vi "Show Animated Busy Icon with Message.vi"(4 "Animated Busy Icon Control Name (Animated Busy Icon)":string="Animated Busy Icon", 5 "Already active? (F)":bool, 6 "Message Control Name (Message)":string="Message", 7 "Message":string, 9 "Error In":errorcluster, 11 "Target VI reference":refnum<vi>) -> (1 "Error Out":errorcluster)   [LabVIEW 2019]
doc: "This VI passes error in through and ignores it"
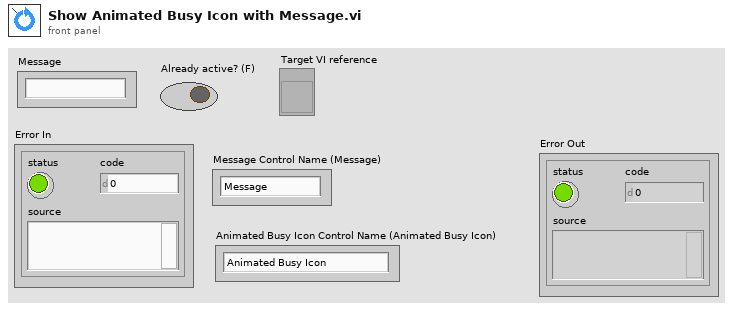
[diagram p1: front panel]
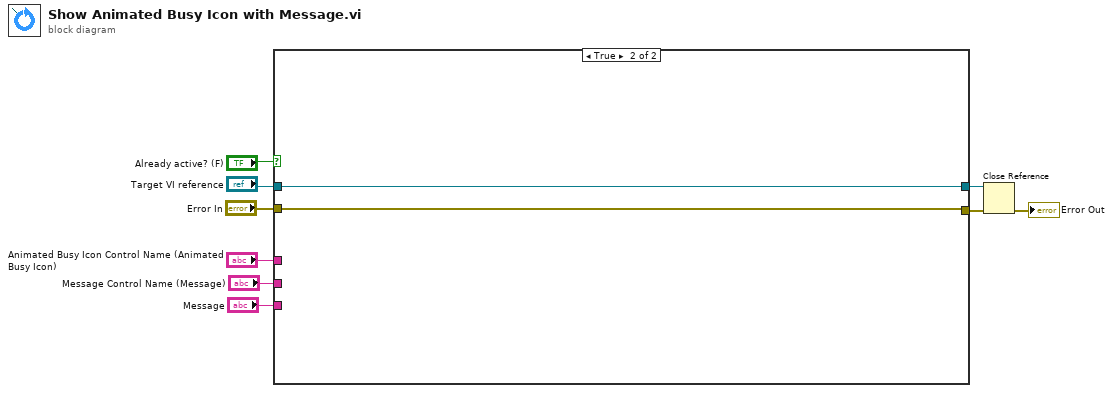
[diagram p0: block diagram]
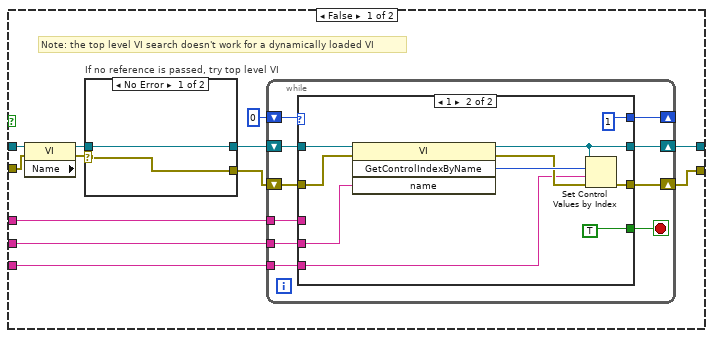
[diagram p2: hidden frame]
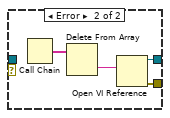
[diagram p3: hidden frame]
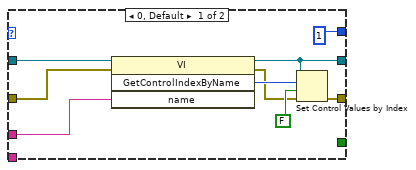
[diagram p4: hidden frame]
diagram:
  n1 = case shown="True" "Already active? (F)" {
    tunnel: [w19 w58] -> w9
    tunnel: [w18 w57] -> w8
    tunnel: "Message Control Name (Message)" -> [w16 _]
    tunnel: "Animated Busy Icon Control Name (Animated Busy Icon)" -> [w15 _]
    tunnel: "Message" -> [w14 _]
    tunnel: "Target VI reference" -> [w13 w58]
    tunnel: "Error In" -> [w10 w57]
    frame False {
      # "Note: the top level VI search doesn't work for a dynamically loaded VI"
      n2 = property class="VI" props=["Name"](reference=w13, error in=w10) -> (reference out=w11:refnum<vi>, error out=w12:errorcluster)  [unwired: 1 out]
      n3 = case "If no reference is passed, try top level VI" shown="No Error" w12 {
        selector: w12 -> [w22 _]
        tunnel: [w22 w27] -> w21
        tunnel: [w23 w26] -> w20
        tunnel: w11 -> [w23 _]
        frame No Error {
        }
        frame Error {
          n4 = Call Chain() -> (call chain=w24:string[])
          n5 = Delete From Array(array=w24) -> (deleted portion=w25:string)  [unwired: 2 in, 1 out]
          n6 = Open VI Reference(vi path=w25) -> (vi reference=w26:refnum<vi>, error out=w27:errorcluster)  [unwired: 5 in]
        }
      }
      n7 = while {
        shift-right: [w34] -> w18
        shift-left: w21 -> [w37]
        shift-right: [w35] -> w19
        shift-left: w20 -> [w36]
        shift-right: [w32] -> _
        shift-left: 0 -> [w33]
        tunnel: w16 -> [w30]
        tunnel: w15 -> [w29]
        tunnel: w14 -> [w28]
        stop <- w31 stop-if-true
        n8 = case shown="1" w33 {
          tunnel: w37 -> [w43 w54]
          tunnel: w36 -> [w42 w53]
          tunnel: [w41 w52] -> w35
          tunnel: [w40 w51] -> w34
          tunnel: [1 1] -> w32
          tunnel: [_ TRUE] -> w31
          tunnel: w30 -> [_ w48]
          tunnel: w29 -> [w38 _]
          tunnel: w28 -> [_ w47]
          frame 0, Default {
            n9 = invoke class="VI" method="GetControlIndexByName"(reference=w42, error in=w43, "name"=w38) -> (reference out=w41:refnum<vi>, error out=w44:errorcluster, "GetControlIndexByName"=w46:i32)  [unwired: 1 in, 1 out]
            n10 = Set Control Values by Index(0:w41, 1:w46, 2:FALSE ("Visible"), 3:w44) -> (11:w40:errorcluster)
          }
          frame 1 {
            n11 = invoke class="VI" method="GetControlIndexByName"(reference=w53, error in=w54, "name"=w48) -> (reference out=w52:refnum<vi>, error out=w55:errorcluster, "GetControlIndexByName"=w56:i32)  [unwired: 1 in, 1 out]
            n12 = Set Control Values by Index(0:w52, 1:w56, 2:w47, 3:w55) -> (11:w51:errorcluster)
          }
        }
      }
    }
    frame True {
    }
  }
  n13 = Close Reference(reference=w9, error in (no error)=w8) -> (error out=→"Error Out":errorcluster)
